vi "Save XML File (Pretty Format).vi"(8 "error in (no error)":errorcluster, 9 "overwrite file (True)":bool=TRUE, 10 "XML file path":path, 11 "DOM document in":refnum<k20>) -> (0 "error out":errorcluster, 2 "XML file path out":path, 3 "DOM document out":refnum<k20>)   [LabVIEW 2017, in "Error File Management.lvlib"]
uses:
  Error File Management.lvlib
  <vilib>/Utility/error.llb/Error Cluster From Error Code.vi
  <vilib>/ErrorRing/Error Ring.xnode
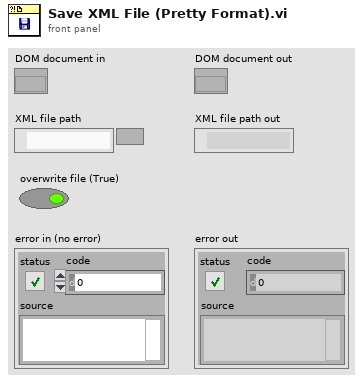
[diagram p1: front panel]
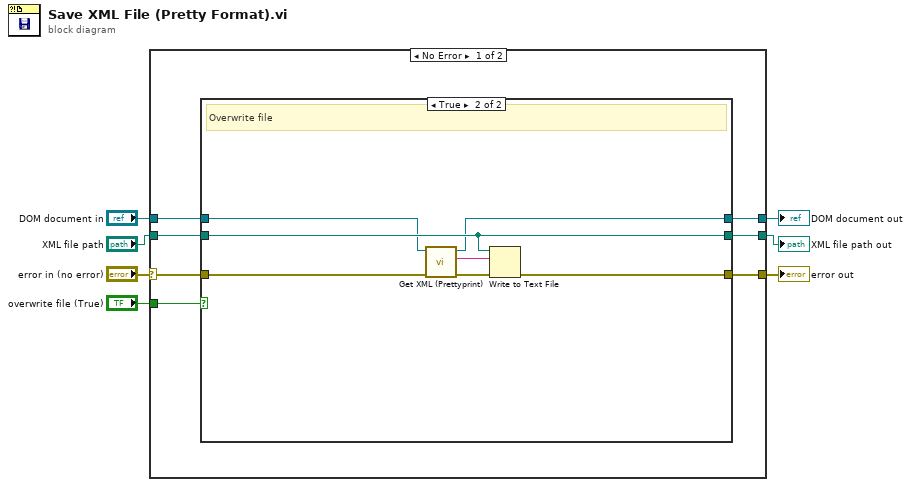
[diagram p0: block diagram]
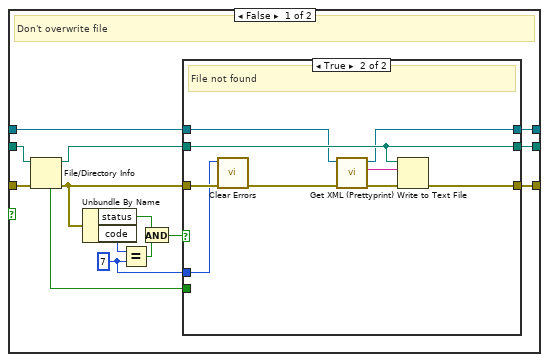
[diagram p2: hidden frame]
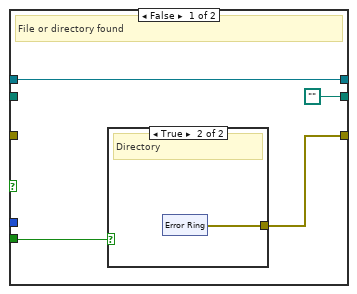
[diagram p3: hidden frame]
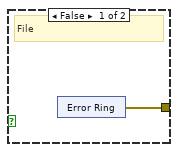
[diagram p4: hidden frame]
diagram:
  n1 = case shown="No Error" "error in (no error)" {
    selector: "error in (no error)" -> [w9 w61]
    tunnel: [w14 w61] -> w3
    tunnel: [w13 w59] -> w7
    tunnel: "DOM document in" -> [w12 w60]
    tunnel: "XML file path" -> [w11 w59]
    tunnel: [w10 w60] -> w1
    tunnel: "overwrite file (True)" -> [w8 _]
    frame No Error {
      n2 = case shown="True" w8 {
        tunnel: w11 -> [w28 w57]
        tunnel: w12 -> [w21 w55]
        tunnel: [w20 w58] -> w14
        tunnel: [w19 w57] -> w13
        tunnel: [w18 w56] -> w10
        tunnel: w9 -> [w17 w54]
        frame False {
          w15 = 7 ("y")
          # "Don't overwrite file"
          n3 = File/Directory Info(path=w28, error in=w17) -> (path out=w27:path, directory=w26:bool, error out=w16:errorcluster)  [unwired: 4 out]
          n4 = Unbundle By Name(w16) -> ("status"=w23:bool, "code"=w25:i32)
          n5 = Equal?(x=w25, y=w15) -> (x = y?=w22:bool)
          n6 = And(x=w23, y=w22) -> (x .and. y?=w24:bool)
          n7 = case shown="True" w24 {
            tunnel: w27 -> [_ w50]
            tunnel: w26 -> [w32 _]
            tunnel: w21 -> [w29 w49]
            tunnel: [w31 w51] -> w20
            tunnel: [path "" w50] -> w19
            tunnel: [w29 w48] -> w18
            tunnel: w16 -> [_ w47]
            tunnel: w15 -> [_ w46]
            frame False {
              # "File or directory found"
              n8 = case shown="True" w32 {
                tunnel: [w33 w38] -> w31
                frame False {
                  # "File"
                  n9 = xnode "Error Ring"() -> ("error out"=w33:errorcluster)
                }
                frame True {
                  # "Directory"
                  n10 = xnode "Error Ring"() -> ("error out"=w38:errorcluster)
                }
              }
            }
            frame True {
              # "File not found"
              n11 = call <vilib>:"Clear Errors.vi"("error in (no error)"=w47, "specific error code to clear (0: all)"=w46) -> ("error out"=w45:errorcluster)  [unwired: 4 in, 1 out]
              n12 = call "Get XML (Prettyprint).vi"("error in (no error)"=w45, "DOM document in"=w49) -> ("error out"=w44:errorcluster, "pretty formatted XML"=w43:string, "DOM document out"=w48:refnum<k20>)  [unwired: 7 in]
              n13 = Write to Text File(file (use dialog)=w50, text=w43, error in=w44) -> (error out=w51:errorcluster)  [unwired: 1 in, 2 out]
            }
          }
        }
        frame True {
          # "Overwrite file"
          n14 = call "Get XML (Prettyprint).vi"("error in (no error)"=w54, "DOM document in"=w55) -> ("error out"=w53:errorcluster, "pretty formatted XML"=w52:string, "DOM document out"=w56:refnum<k20>)  [unwired: 7 in]
          n15 = Write to Text File(file (use dialog)=w57, text=w52, error in=w53) -> (error out=w58:errorcluster)  [unwired: 1 in, 2 out]
        }
      }
    }
    frame Error {
    }
  }
  "XML file path out" <- w7
  "error out" <- w3
  "DOM document out" <- w1
